vi "main.vi"() -> ()   [LabVIEW 2020]
doc: "Ce VI modèle est conçu pour le modèle de conception Gestionnaire de messages dans une file d'attente.\n\nLa boucle de gestion d'événements génère des messages en fonction des actions sur l'interface utilisateur.\n\nLa boucle de gestion de messages traite les messages générés par la boucle de gestion d'événements ou par d'autres messages. Les messages sont des valeurs chaîne ; il est donc facile d'ajouter de nouveaux messages à la structure condition Conditions de messages de la boucle de gestion de messages Chaque cluster Message peut en outre fournir une valeur optionnelle pour Données de message, un variant qui peut être converti aux données requises pour un message spécifique."
uses:
  controls/UI Data.ctl
  support/Message Queue/Enqueue Message (Single).vi
  <vilib>/Utility/error.llb/Error Cluster From Error Code.vi
  <vilib>/ErrorRing/Error Ring.xnode
  support/Message Queue/Message Queue.lvlib
  support/User Event - Stop/User Event - Stop.lvlib
  cDaqlib/cDaq.lvlib
panel:
  in  "Target position(°)":dbl
  in  "frequency (Hz)":i32 min=0 max=4000 step=1
  out "isHome?":bool
  in  "Tourner vers position":bool
  in  "Tourner en continue":bool
  out "ms for 1°":dbl
  out "passed ms":u32
  out "Position(°)":dbl
  out "AvgTimePerRev(s)":dbl
  out "temps(s)/tour (360°)":dbl[](array[numeric])
  in  "direction":bool
  out "enable = 0":i32
  out "tension compteur (V)":dbl
  out "DAQ HANDLE":u32
  out "Exit":bool
  out "compteur":i32
  out "Rotation status":bool
  in  "calibrer":bool
  in  "adresse":string
  out "Debug":string
  in  "deconnecter":bool
  in  "connecter":bool
  in  "Quitter":bool
  # "D'abord se connecter par USB à la carte DAQ. Si pas de nom préscisé le premier équipement disponible sera choisis."
  # "Passage devant\ndétecteur"
  # "Ferme proprement la connection avec la carte et libère les ressources."
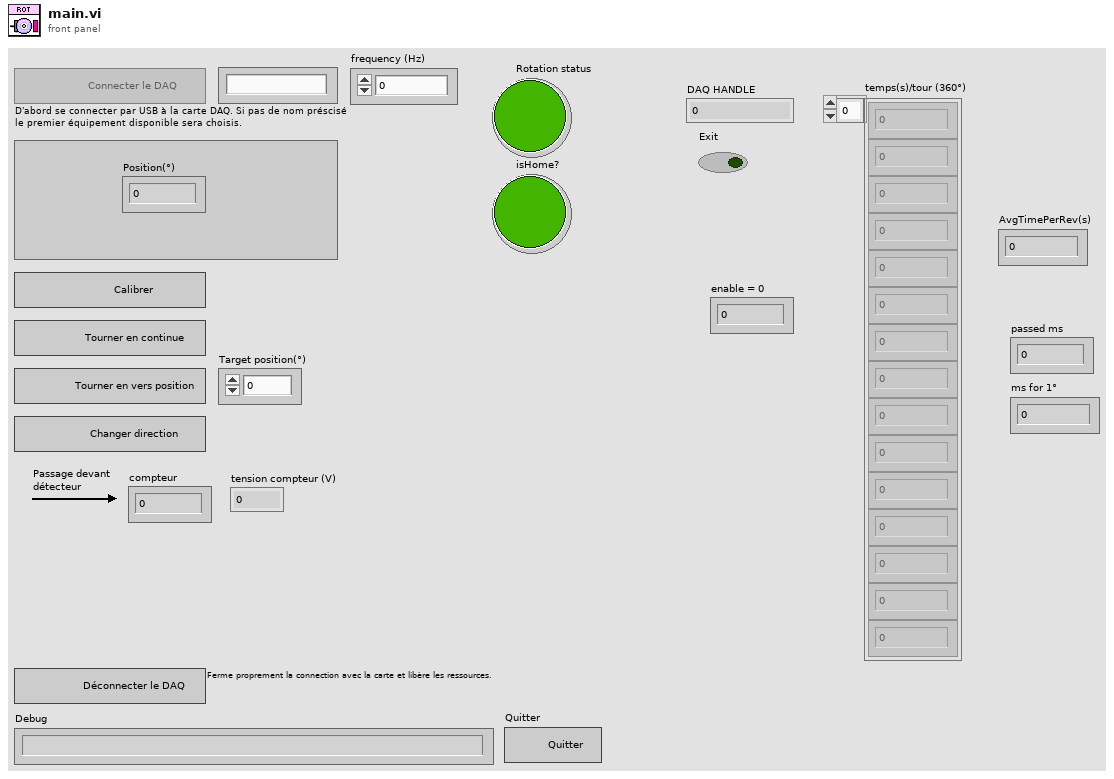
[diagram p1: front panel]
types:
  T1 = typedef "UI Data.ctl" = cluster{"Booléen <À remplacer>":bool, "Chaîne <À remplacer>":string, "Numérique <À remplacer>":dbl, "Réf. Action 1":refnum<vi>, "Réf. Action 2":refnum<vi>, "Réf. Affichage des données":refnum<vi>, "Réf du bouton Quitter":refnum<vi>, "DAQ handle":u32, "DAQ HANDLE ref":refnum<vi>, "frequency":refnum<vi>, "status":refnum<vi>, "Position(°)":refnum<vi>, "isHome?":refnum<vi>}
  T2 = cluster{"état":bool, "code":i32, "source":string}
  T3 = typedef "Message Queue.lvlib/All Message Queues.ctl" = cluster{"IU":refnum<queue>}
  T4 = enum8{"Enabled", "Disabled", "Disabled and Grayed Out"}
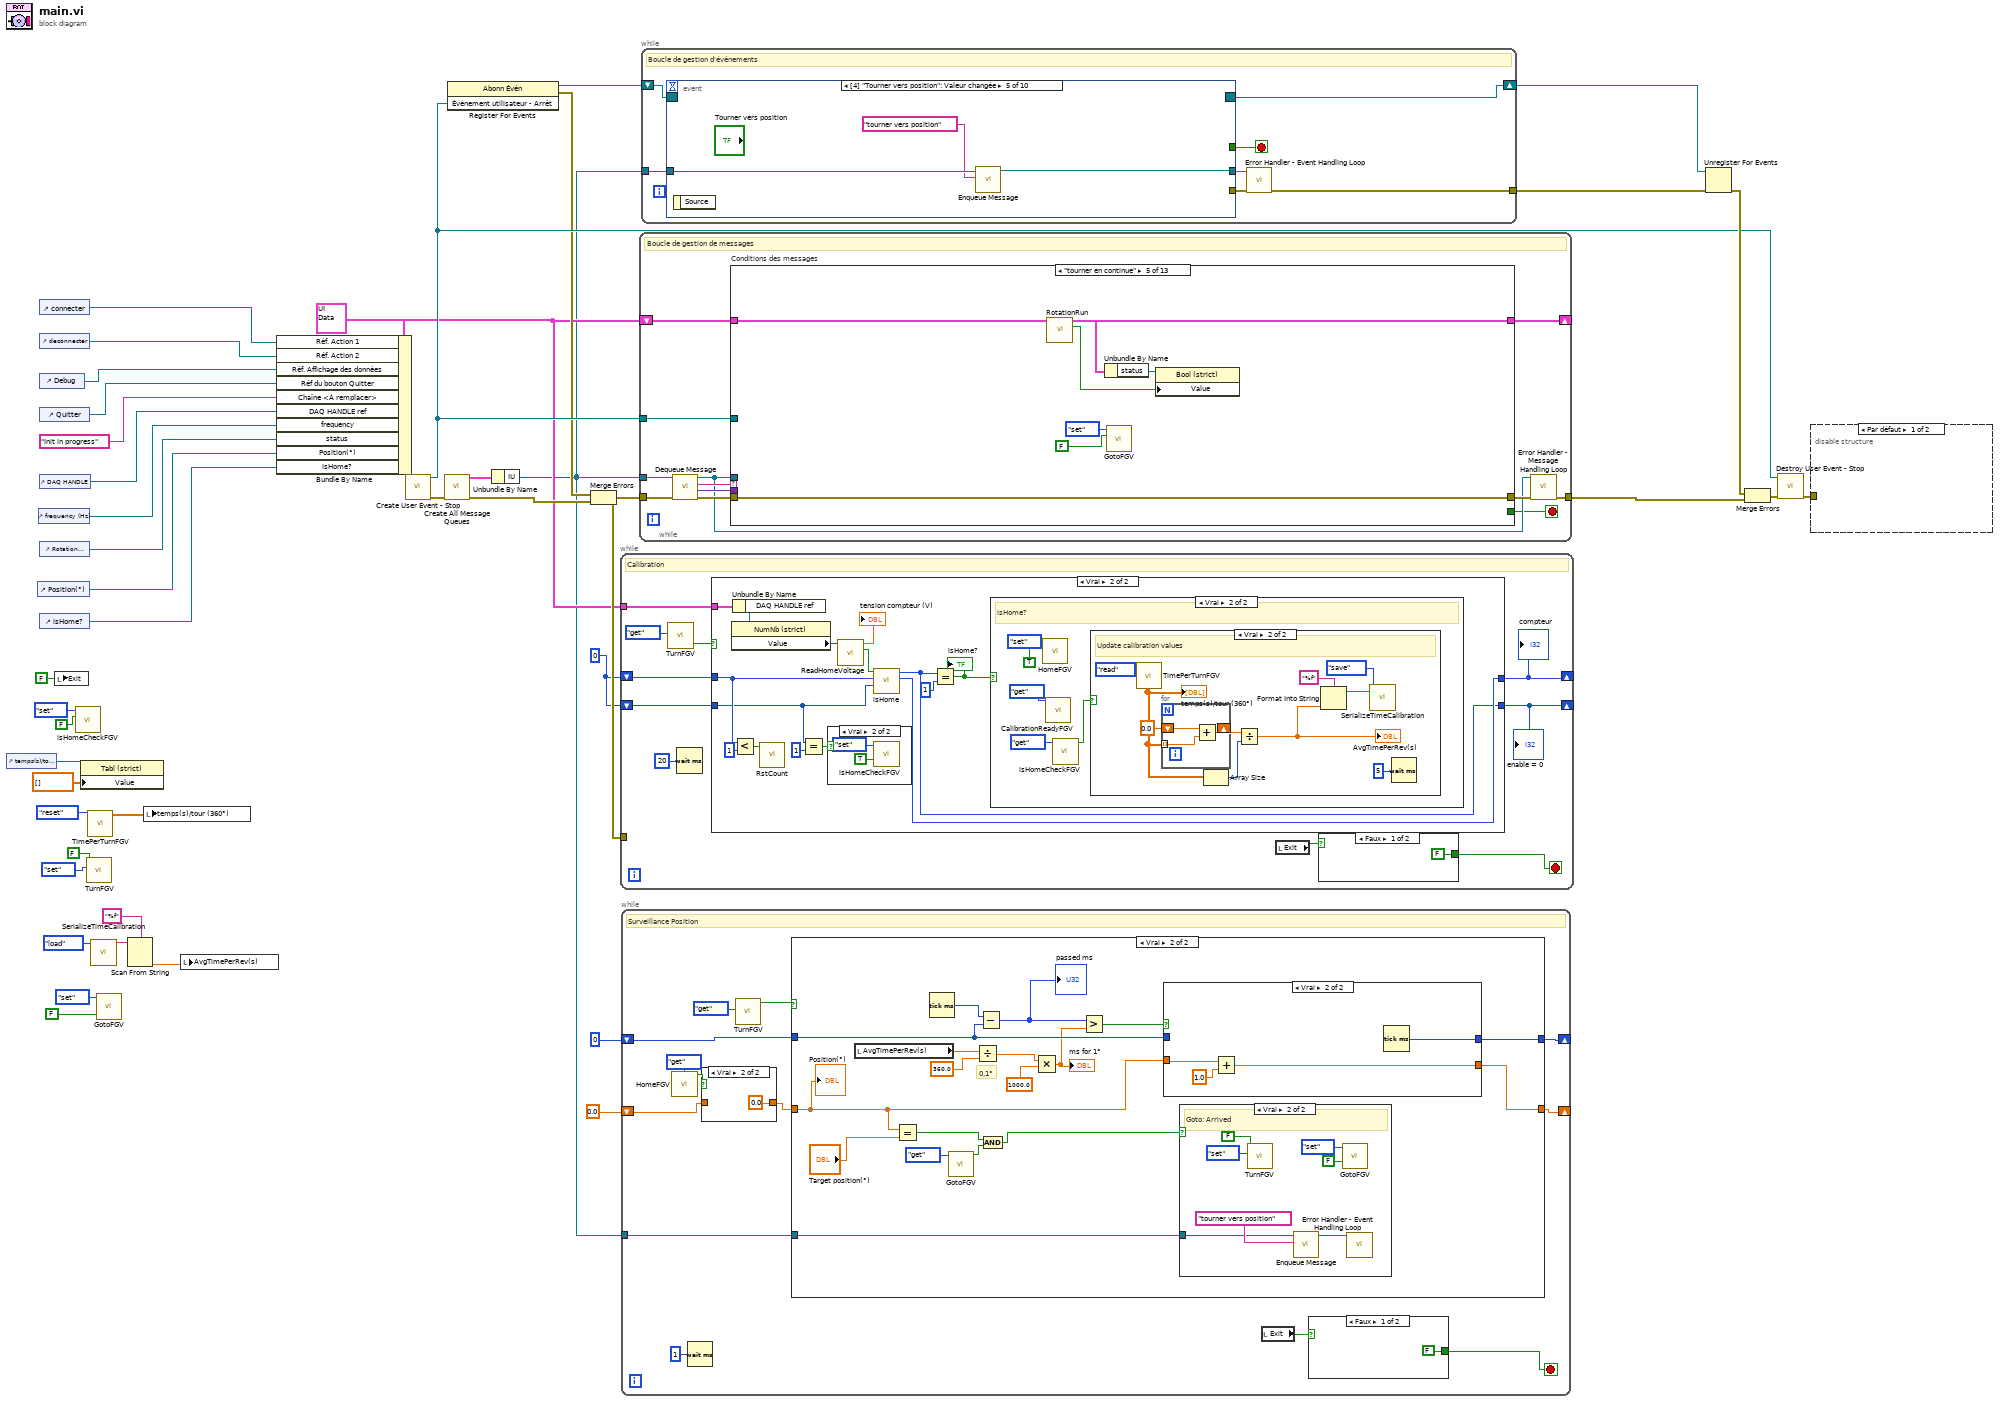
[diagram p0: block diagram]
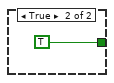
[diagram p3: hidden frame]
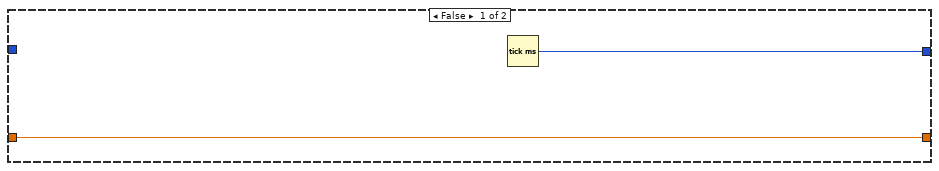
[diagram p4: hidden frame]
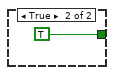
[diagram p7: hidden frame]
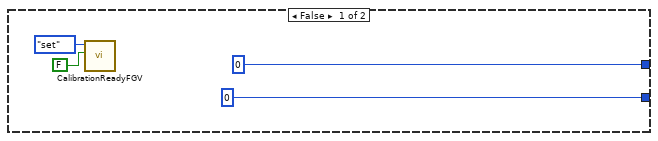
[diagram p8: hidden frame]
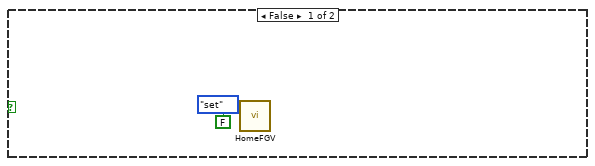
[diagram p10: hidden frame]
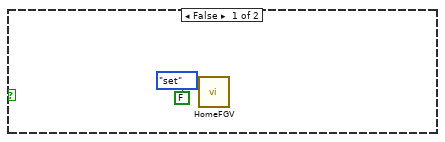
[diagram p11: hidden frame]
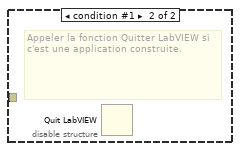
[diagram p12: hidden frame]
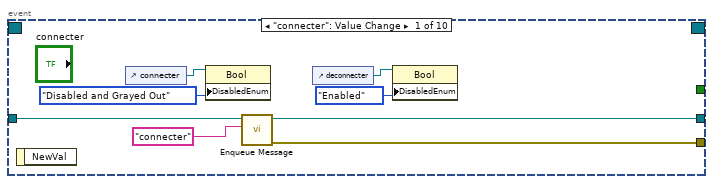
[diagram p13: hidden frame]
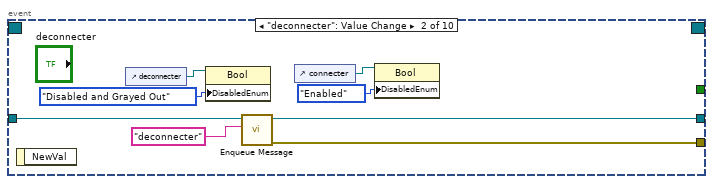
[diagram p14: hidden frame]
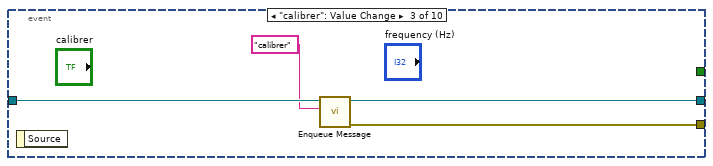
[diagram p15: hidden frame]
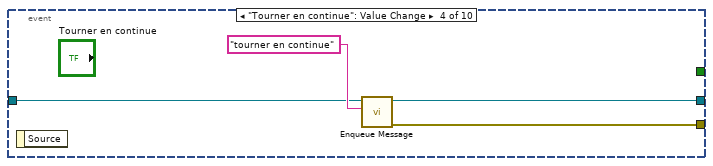
[diagram p16: hidden frame]
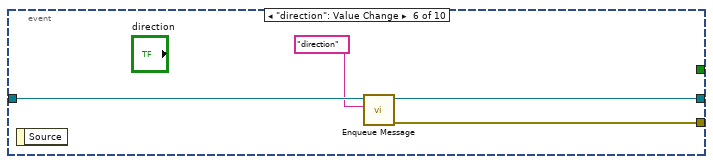
[diagram p17: hidden frame]
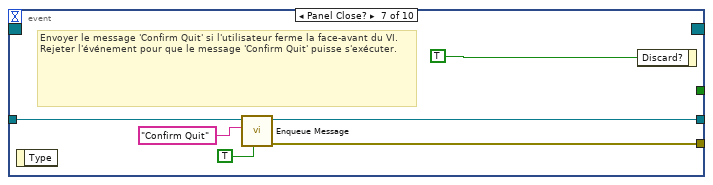
[diagram p18: hidden frame]
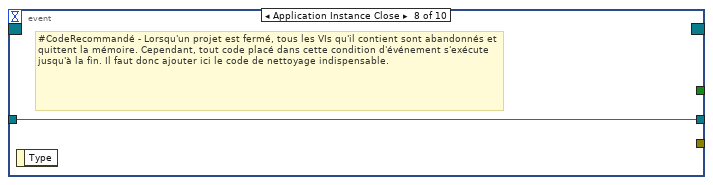
[diagram p19: hidden frame]
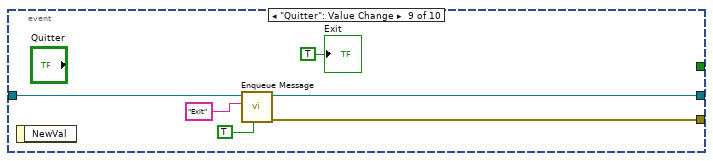
[diagram p20: hidden frame]
diagram:
  w22 = 0
  n1 = control-ref of="temps(s)/tour (360°)"() -> (w19:refnum<vi>)
  n2 = control-ref of="Position(°)"() -> (w9:refnum<vi>)
  n3 = control-ref of="frequency (Hz)"() -> (w4:refnum<vi>)
  n4 = control-ref of="connecter"() -> (w29:refnum<vi>)
  n5 = control-ref of="deconnecter"() -> (w30:refnum<vi>)
  n6 = control-ref of="Debug"() -> (w31:refnum<vi>)
  n7 = control-ref of="Quitter"() -> (w7:refnum<vi>)
  n8 = control-ref of="DAQ HANDLE"() -> (w10:refnum<vi>)
  n9 = control-ref of="Rotation status"() -> (w11:refnum<vi>)
  n10 = control-ref of="isHome?"() -> (w8:refnum<vi>)
  n11 = local write "Exit"(FALSE ("Exit")) -> ()
  n12 = call "isHomeCheckFGV.vi"("isHomeCheck?"=FALSE, "state"=enum16{"get", "set"}."set") -> ()  [unwired: 9 in, 1 out]
  n13 = property class="Tabl (strict)"(reference=w19, "Value"=dbl[] [] ("Valeur")) -> ()  [unwired: 1 in, 2 out]
  n14 = call "TurnFGV.vi"("Énum"=enum16{"set", "get"}."set", "set"=FALSE) -> ()  [unwired: 9 in, 1 out]
  n15 = call "TimePerTurnFGV.vi"("Énum"=enum16{"reset", "read", "home"}."reset") -> ("temps(s)/tour (360°)"=w16:dbl[])  [unwired: 9 in, 1 out]
  n16 = call "SerializeTimeCalibration.vi"("cmd"=enum16{"load", "save"}."load") -> ("TimeCalibration out"=w15:string)  [unwired: 10 in]
  n17 = call "GotoFGV.vi"("goto?"=FALSE, "goto pos"=enum16{"get", "set"}."set") -> ()  [unwired: 9 in, 1 out]
  n18 = Scan From String(format string="%f" ("chaîne de format"), input string=w15) -> (output 1=w12:dbl)  [unwired: 3 in, 3 out]
  n19 = local write "temps(s)/tour (360°)"(w16) -> ()
  n20 = local write "AvgTimePerRev(s)"(w12) -> ()
  n21 = Bundle By Name(cluster=T1 {"Booléen <À remplacer>"=FALSE, "Chaîne <À remplacer>"="", "Numérique <À remplacer>"=0.0, "Réf. Action 1"=refnum, "Réf. Action 2"=refnum, "Réf. Affichage des données"=refnum, "Réf du bouton Quitter"=refnum, "DAQ handle"=0, "DAQ HANDLE ref"=refnum, "frequency"=refnum, "status"=refnum, "Position(°)"=refnum, "isHome?"=refnum} ("Data Cluster"), "Réf. Action 1"=w29, "Réf. Action 2"=w30, "Réf. Affichage des données"=w31, "Réf du bouton Quitter"=w7, "Chaîne <À remplacer>"="Init in progress" ("Initial Message"), "DAQ HANDLE ref"=w10, "frequency"=w4, "status"=w11, "Position(°)"=w9, "isHome?"=w8) -> (w26:T1)
  n22 = call "Create User Event - Stop.vi"() -> ("error out"=w41:T2, "Événement utilisateur - Arrêt"=w34:refnum<user-event>)  [unwired: 10 in]
  n23 = call "Create All Message Queues.vi"("error in (no error)"=w41) -> ("error out"=w44:T2, "Files d'attente de messages en sortie"=w43:T3)  [unwired: 9 in]
  n24 = register-events(w34) -> (reference out=w35:refnum<event-registration>, error out=w33:errorcluster)  [unwired: 2 in]
  n25 = Unbundle By Name(w43) -> ("IU"=w1:refnum<queue>)
  n26 = Merge Errors(w33, w44) -> (w32:errorcluster)
  n27 = while {
    tunnel: w26 -> [w47]
    shift-right: [w50] -> _
    shift-left: w22 -> [w51]
    tunnel: w32 -> [_]
    shift-right: [w45] -> _
    shift-left: w22 -> [w46]
    stop <- w49 stop-if-true
    # "Calibration"
    n28 = call "TurnFGV.vi"("Énum"=enum16{"set", "get"}."get") -> ("get"=w53:bool)  [unwired: 10 in]
    n29 = Wait (ms)(milliseconds to wait=u32 20 ("attente (ms)")) -> ()  [unwired: 1 out]
    n30 = case shown="Vrai" w53 {
      tunnel: w47 -> [_ w75]
      tunnel: w51 -> [_ w62]
      tunnel: [0 w72] -> w50
      tunnel: w46 -> [_ w61]
      tunnel: [0 w65] -> w45
      frame False {
        n31 = call "CalibrationReadyFGV.vi"("Énum"=enum16{"get", "1stClk", "set"}."set", "set"=FALSE) -> ()  [unwired: 8 in, 1 out]
      }
      frame True {
        n32 = Unbundle By Name(w75) -> ("DAQ HANDLE ref"=w71:refnum<vi>)
        n33 = property class="NumNb (strict)"(reference=w71) -> ("Value"=w70:u32)  [unwired: 1 in, 2 out]
        n34 = Less?(x=w62, y=1) -> (x < y?=w67:bool)
        n35 = call "RstCount.vi"("Reset counter"=w67) -> ()  [unwired: 11 in]
        n36 = Equal?(x=w61, y=1) -> (x = y?=w63:bool)
        n37 = case shown="Vrai" w63 {
          frame False {
          }
          frame True {
            n38 = call "isHomeCheckFGV.vi"("isHomeCheck?"=TRUE, "state"=enum16{"get", "set"}."set") -> ()  [unwired: 9 in, 1 out]
          }
        }
        n39 = call "ReadHomeVoltage.vi"("Handle"=w70) -> ("At home"=w73:bool, "Voltage read 0V=in position"=→"tension compteur (V)":dbl)  [unwired: 9 in]
        n40 = call "isHome.vi"("HomeDetected last state"=w61, "Counter last state"=w62, "Home area detected"=w73) -> ("Counter"=w72:i32, "HomeDetected=1"=w65:i32)  [unwired: 7 in]
        n41 = Equal?(x=w65, y=1) -> (x = y?=w64:bool)
        "isHome?" <- w64
        n42 = case shown="Vrai" w64 {
          frame False {
            n43 = call "HomeFGV.vi"("Énum"=enum16{"set", "get"}."set", "Booléen"=FALSE) -> ()  [unwired: 8 in, 1 out]
          }
          frame True {
            # "isHome?"
            n44 = call "HomeFGV.vi"("Énum"=enum16{"set", "get"}."set", "Booléen"=TRUE) -> ()  [unwired: 8 in, 1 out]
            n45 = call "CalibrationReadyFGV.vi"("Énum"=enum16{"get", "1stClk", "set"}."get") -> ()  [unwired: 9 in, 1 out]
            n46 = call "isHomeCheckFGV.vi"("state"=enum16{"get", "set"}."get") -> ("HomeisCheck"=w81:bool)  [unwired: 10 in]
            n47 = case shown="Vrai" w81 {
              frame False {
                n48 = call "HomeFGV.vi"("Énum"=enum16{"set", "get"}."set", "Booléen"=FALSE) -> ()  [unwired: 8 in, 1 out]
              }
              frame True {
                # "Update calibration values"
                n49 = call "TimePerTurnFGV.vi"("Énum"=enum16{"reset", "read", "home"}."read") -> ("temps(s)/tour (360°)"=w95:dbl[])  [unwired: 9 in, 1 out]
                "temps(s)/tour (360°)" <- w95
                n50 = for {
                  tunnel: w95 -> [w98] mode=indexing
                  shift-right: [w97] -> w94
                  shift-left: 0.0 -> [w99]
                  n51 = Add(x=w99, y=w98) -> (x+y=w97:dbl)
                }
                n52 = Array Size(array=w95) -> (size(s)=w93:i32)
                n53 = Divide(x=w94, y=w93) -> (x/y=w88:dbl)
                "AvgTimePerRev(s)" <- w88
                n54 = Format Into String(format string="%f" ("chaîne de format"), w88) -> (resulting string=w89:string)  [unwired: 2 in, 1 out]
                n55 = call "SerializeTimeCalibration.vi"("TimeCalibration in"=w89, "cmd"=enum16{"load", "save"}."save") -> ()  [unwired: 9 in, 1 out]
                n56 = Wait (ms)(milliseconds to wait=u32 5 ("attente (ms)")) -> ()  [unwired: 1 out]
              }
            }
          }
        }
      }
    }
    "compteur" <- w50
    "enable = 0" <- w45
    n57 = local read "Exit"() -> (w48:bool)
    n58 = case shown="Faux" w48 {
      tunnel: [FALSE TRUE] -> w49
      frame False {
      }
      frame True {
      }
    }
  }
  n59 = while {
    shift-right: [w109] -> _
    shift-left: u32 0 ("millisecond timer value") -> [w112]
    shift-right: [w108] -> _
    shift-left: 0.0 -> [w104]
    tunnel: w1 -> [w100]
    stop <- w111 stop-if-true
    # "Surveillance Position"
    n60 = call "HomeFGV.vi"("Énum"=enum16{"set", "get"}."get") -> ("home ?"=w106:bool)  [unwired: 9 in]
    n61 = Wait (ms)(milliseconds to wait=u32 1 ("attente (ms)")) -> ()  [unwired: 1 out]
    n62 = case shown="Vrai" w106 {
      tunnel: w104 -> [w113 _]
      tunnel: [w113 0.0] -> w103
      frame False {
      }
      frame True {
      }
    }
    n63 = call "TurnFGV.vi"("Énum"=enum16{"set", "get"}."get") -> ("get"=w101:bool)  [unwired: 10 in]
    n64 = case shown="Vrai" w101 {
      tunnel: w112 -> [_ w131]
      tunnel: [w118 w130] -> w109
      tunnel: w103 -> [w117 w125]
      tunnel: [w117 w132] -> w108
      tunnel: w100 -> [_ w119]
      frame False {
        n65 = Tick Count (ms)() -> (millisecond timer value=w118:u32)
      }
      frame True {
        # "0,1°"
        n66 = local read "AvgTimePerRev(s)"() -> (w135:dbl)
        n67 = Equal?(x=w125, y="Target position(°)") -> (x = y?=w123:bool)
        n68 = Tick Count (ms)() -> (millisecond timer value=w136:u32)
        n69 = call "GotoFGV.vi"("goto pos"=enum16{"get", "set"}."get") -> ("moving to position"=w121:bool)  [unwired: 10 in]
        n70 = Divide(x=w135, y=360.0) -> (x/y=w129:dbl)
        n71 = Subtract(x=w136, y=w131) -> (x-y=w126:u32)
        "passed ms" <- w126
        n72 = And(x=w123, y=w121) -> (x .and. y?=w120:bool)
        n73 = Multiply(x=w129, y=1000.0) -> (x*y=w127:dbl)
        "ms for 1°" <- w127
        n74 = Greater?(x=w126, y=w127) -> (0:w133:bool)
        n75 = case shown="Vrai" w133 {
          tunnel: w125 -> [w145 w149]
          tunnel: [w145 w146] -> w132
          tunnel: w131 -> [w144 _]
          tunnel: [w144 w147] -> w130
          frame False {
          }
          frame True {
            n76 = Add(x=w149, y=1.0) -> (x+y=w146:dbl)
            n77 = Tick Count (ms)() -> (millisecond timer value=w147:u32)
          }
        }
        n78 = case shown="Vrai" w120 {
          tunnel: w119 -> [_ w137]
          frame False {
          }
          frame True {
            # "Goto: Arrived"
            n79 = call "TurnFGV.vi"("Énum"=enum16{"set", "get"}."set", "set"=FALSE) -> ()  [unwired: 9 in, 1 out]
            n80 = call-poly "Enqueue Message.vi"("Message"="tourner vers position", "File d'attente de messages"=w137) -> ("File d'attente de message dup."=w139:refnum<queue>)  [unwired: 8 in, 1 out]
            n81 = call "GotoFGV.vi"("goto?"=FALSE, "goto pos"=enum16{"get", "set"}."set") -> ()  [unwired: 9 in, 1 out]
            n82 = call "Error Handler - Event Handling Loop.vi"("File d'attente de messages"=w139) -> ()  [unwired: 9 in, 2 out]
          }
        }
        "Position(°)" <- w125
      }
    }
    n83 = local read "Exit"() -> (w110:bool)
    n84 = case shown="Faux" w110 {
      tunnel: [FALSE TRUE] -> w111
      frame False {
      }
      frame True {
      }
    }
  }
  n85 = while {
    tunnel: w1 -> [w154]
    shift-right: [w160] -> _
    shift-left: w26 -> [w161]
    tunnel: w34 -> [w159]
    tunnel: w32 -> [w158]
    tunnel: [w153] -> w42
    stop <- w150 stop-if-true
    # "Boucle de gestion de messages"
    n86 = call "Dequeue Message.vi"("error in (no error)"=w158, "File d'attente de messages"=w154) -> ("error out"=w157:T2, "Données de message"=w155:variant, "Message"=w156:string, "File d'attente de message dup."=w151:refnum<queue>)  [unwired: 6 in]
    n87 = case "Conditions des messages" shown="\"tourner en continue\"" w156 {
      selector: w156 -> [_ _ _ _ _ _ _ _ _ _ _ _ w289]
      tunnel: w151 -> [w176 w191 w212 _ _ _ _ _ _ w263 _ w287 _]
      tunnel: w157 -> [w178 w192 w214 w224 w231 w238 w246 w251 w260 w267 w270 w281 _]
      tunnel: [w179 w193 w215 w224 w231 w238 w246 w252 w254 w265 w268 w284 w290] -> w152
      tunnel: w161 -> [w168 w180 w207 w220 w230 w236 w245 w253 w259 w266 w269 w274 w291]
      tunnel: [w168 w181 w207 w222 w227 w234 w245 w253 w259 w266 w269 w274 w291] -> w160
      tunnel: [_ _ _ _ _ _ _ _ _ _ _ TRUE _] -> w150
      tunnel: w155 -> [_ _ _ _ _ _ _ w250 w258 _ _ w278 _]
      tunnel: w159 -> [_ _ _ _ _ _ _ _ _ _ _ w283 _]
      frame "Initialize" {
        # "Initialize - Toute la tâche d'initialisation doit se faire dans ce message puisque les autres boucles risquent d'ajouter des messages qui s'exécutent juste après celui-ci à la file."
        n88 = control-ref of="Rotation status"() -> (w175:refnum<vi>)
        n89 = control-ref of="connecter"() -> (w173:refnum<vi>)
        n90 = control-ref of="deconnecter"() -> (w174:refnum<vi>)
        n91 = property class="Bool (strict)"(reference=w175, "DisabledEnum"=T4."Disabled" ("Désactivé")) -> ()  [unwired: 1 in, 2 out]
        n92 = property class="Bool"(reference=w173, "DisabledEnum"=T4."Enabled" ("Désactivé")) -> ()  [unwired: 1 in, 2 out]
        n93 = property class="Bool"(reference=w174, "DisabledEnum"=T4."Disabled and Grayed Out" ("Désactivé")) -> ()  [unwired: 1 in, 2 out]
        n94 = Unbundle By Name(w168) -> ("status"=w167:refnum<vi>, "isHome?"=w164:refnum<vi>, "DAQ HANDLE ref"=w163:refnum<vi>)
        n95 = call-poly "Enqueue Message.vi"("error in (no error)"=w178, "Données de message"="initialize" ("Message"), "Message"="Update Display", "File d'attente de messages"=w176) -> ("error out"=w179:T2)  [unwired: 6 in, 1 out]
        n96 = property class="NumNb (strict)"(reference=w163, "Value"=u32 0 ("Valeur")) -> ()  [unwired: 1 in, 2 out]
        n97 = property class="Bool (strict)"(reference=w167, "Value"=FALSE ("Valeur")) -> ()  [unwired: 1 in, 2 out]
        n98 = property class="Bool (strict)"(reference=w164, "Value"=FALSE ("Valeur")) -> ()  [unwired: 1 in, 2 out]
      }
      frame "connecter" {
        w186 = "Update Display" ("Message")
        # "Appel la DLL pour se connecter au DAQ"
        n99 = call "createDAQ.vi"("device"="adresse") -> ("function return"=w184:u32)  [unwired: 9 in]
        "DAQ HANDLE" <- w184
        n100 = call-poly "Enqueue Message.vi"("error in (no error)"=w192, "Données de message"="Demande de connection" ("\"Do Something\" button pressed"), "Message"=w186, "File d'attente de messages"=w191) -> ("error out"=w188:T2, "File d'attente de message dup."=w189:refnum<queue>)  [unwired: 6 in]
        n101 = Not Equal?(x=w184, y=u32 0) -> (x != y?=w182:bool)
        n102 = case shown="Vrai" w182 {
          tunnel: w189 -> [_ w203]
          tunnel: w188 -> [_ w202]
          tunnel: [T2 {"état"=TRUE, "code"=0, "source"="Erreur de connection"} ("error out") w201] -> w187
          tunnel: w186 -> [_ w200]
          tunnel: w180 -> [w195 w198]
          tunnel: w184 -> [_ w197]
          tunnel: [w195 w196] -> w181
          frame False {
          }
          frame True {
            n103 = Bundle By Name(cluster=w198, "DAQ handle"=w197) -> (w196:T1)
            n104 = call-poly "Enqueue Message.vi"("error in (no error)"=w202, "Données de message"="Connecté" ("\"Do Something\" button pressed"), "Message"=w200, "File d'attente de messages"=w203) -> ("error out"=w201:T2)  [unwired: 6 in, 1 out]
          }
        }
        n105 = Merge Errors(w187) -> (w193:errorcluster)
      }
      frame "deconnecter" {
        # "Libère les ressources"
        n106 = Unbundle By Name(w207) -> ("DAQ HANDLE ref"=w206:refnum<vi>)
        n107 = property class="NumNb (strict)"(reference=w206) -> ("Value"=w208:u32)  [unwired: 1 in, 2 out]
        n108 = call "destroyDAQ.vi"("handle"=w208) -> ("Succés?"=w209:bool)  [unwired: 10 in]
        n109 = case shown="Vrai" w209 {
          tunnel: w206 -> [_ w217]
          frame False {
          }
          frame True {
            n110 = property class="NumNb (strict)"(reference=w217, "Value"=u32 0 ("DAQ handle")) -> ()  [unwired: 1 in, 2 out]
          }
        }
        n111 = call-poly "Enqueue Message.vi"("error in (no error)"=w214, "Données de message"="DAQ déconnecté" ("\"Do Something Else\" button pressed"), "Message"="Update Display", "File d'attente de messages"=w212) -> ("error out"=w213:T2)  [unwired: 6 in, 1 out]
        n112 = Merge Errors(w213) -> (w215:errorcluster)
        n113 = call "TurnFGV.vi"("Énum"=enum16{"set", "get"}."set", "set"=FALSE) -> ()  [unwired: 9 in, 1 out]
      }
      frame "calibrer" {
        n114 = call "GotoFGV.vi"("goto?"=FALSE, "goto pos"=enum16{"get", "set"}."set") -> ()  [unwired: 9 in, 1 out]
        n115 = call "RotationRun.vi"("Data Cluster en entrée"=w220) -> ("Booléen"=→"Rotation status":bool, "Data Cluster en sortie"=w222:T1)  [unwired: 9 in]
        n116 = call "CalibrationStart.vi"("Booléen"=TRUE) -> ()  [unwired: 11 in]
      }
      frame "tourner en continue" {
        n117 = call "RotationRun.vi"("Data Cluster en entrée"=w230) -> ("Booléen"=w228:bool, "Data Cluster en sortie"=w227:T1)  [unwired: 9 in]
        n118 = Unbundle By Name(w230) -> ("status"=w229:refnum<vi>)
        n119 = call "GotoFGV.vi"("goto?"=FALSE, "goto pos"=enum16{"get", "set"}."set") -> ()  [unwired: 9 in, 1 out]
        n120 = property class="Bool (strict)"(reference=w229, "Value"=w228) -> ()  [unwired: 1 in, 2 out]
      }
      frame "tourner vers position" {
        n121 = call "GotoFGV.vi"("goto?"=TRUE, "goto pos"=enum16{"get", "set"}."set") -> ()  [unwired: 9 in, 1 out]
        n122 = call "RotationRun.vi"("Data Cluster en entrée"=w236) -> ("Booléen"=w235:bool, "Data Cluster en sortie"=w234:T1)  [unwired: 9 in]
        n123 = Unbundle By Name(w236) -> ("status"=w237:refnum<vi>)
        n124 = property class="Bool (strict)"(reference=w237, "Value"=w235) -> ()  [unwired: 1 in, 2 out]
      }
      frame "direction" {
        # "Inverser à chaque clic"
        n125 = Unbundle By Name(w245) -> ("DAQ HANDLE ref"=w244:refnum<vi>)
        n126 = property class="NumNb (strict)"(reference=w244) -> ("Value"=w240:u32)  [unwired: 1 in, 2 out]
        n127 = feedback #1(TRUE) -> (w241:bool)
        n128 = call "Direction.vi"("pin"=1, "handle"=w240, "Direction?"=w241) -> ()  [unwired: 8 in, 1 out]
        n129 = Not(x=w241) -> (.not. x?=w242:bool)
        n130 = feedback-in #1(w242) -> ()
      }
      frame "Update Display" {
        # "#CodeRecommandé - Pour séparer la boucle de gestion de messages de l'interface utilisateur, envisagez de créer des événements utilisateur (comme l'événement \"Arrêt\" de ce VI) pour envoyer des messages à la boucle de gestion d'événements quand l'interface utilisateur doit être mise à jour."
        # "Update Display - Convertir les données du message en chaîne pour l'afficher dans l'indicateur Affichage des données."
        n131 = Variant To Data(error in=w251, type="", Variant=w250) -> (data=→"Debug":string, error out=w248:errorcluster)
        n132 = Merge Errors(w248) -> (w252:errorcluster)
      }
      frame "Error" {
        # "#CodeRecommandé - Si vous changez le nom de ce message \"Error\" ici, vous devrez aussi le changer dans le VI Check Loop Error.vi."
        # "#CodeRecommandé - Envisagez de créer un système pour enregistrer les erreurs d'une façon ou d'une autre. Ces erreurs sont uniquement destinées aux notifications. La gestion d'erreurs spécifiques devrait se faire dans les conditons de messages qui ont générées l'erreur."
        # "Error - Afficher une boîte de dialogue d'erreur. Ce message est envoyé par les VIs \"Error Handler\" à la fin de l'exécution de chaque boucle de cette application."
        n133 = Variant To Data(error in=w260, type=errorcluster {"status"=FALSE, "code"=0, "source"=""} ("error constant"), Variant=w258) -> (data=w256:errorcluster, error out=w255:errorcluster)
        n134 = call <vilib>:"Simple Error Handler.vi"("error in (no error)"=w256) -> ()  [unwired: 4 in, 5 out]
        n135 = Merge Errors(w255) -> (w254:errorcluster)
      }
      frame "Confirm Quit" {
        # "#CodeNécessaire - Si vous voulez afficher une boîte de dialogue de confirmation (ou un autre message) avant de quitter l'application, placez le code ici. En général, ce message est envoyé à partir d'un événement Fermeture de face-avant ?"
        # "Confirm Quit - Message qui confirme si l'utilisateur voulait vraiment quitter l'application."
        n136 = call-poly "Enqueue Message.vi"("Message prioritaire ? (F)"=TRUE ("Priority Message? (F)"), "error in (no error)"=w267, "Message"="Exit", "File d'attente de messages"=w263) -> ("error out"=w264:T2)  [unwired: 6 in, 1 out]
        n137 = Merge Errors(w264) -> (w265:errorcluster)
      }
      frame "---Copy This Frame---" {
        # "Dupliquez cette étape pour créer de nouveaux messages.  Changez ce commentaire dans l'étape dupliquée pour décrire ce message."
        n138 = Merge Errors(w270) -> (w268:errorcluster)
      }
      frame "Exit" {
        # "Arrêter le VI"
        # "Libérer la référence à la file d'attente de messages"
        # "Exit - Quitter l'application."
        n139 = Unbundle By Name(w274) -> ("DAQ HANDLE ref"=w277:refnum<vi>)
        n140 = Variant To Data(type=errorcluster {"status"=FALSE, "code"=0, "source"=""} ("error constant"), Variant=w278) -> (data=w279:errorcluster)  [unwired: 1 in, 1 out]
        n141 = call <vilib>:"Simple Error Handler.vi"("error in (no error)"=w279) -> ()  [unwired: 4 in, 5 out]
        n142 = call "TurnFGV.vi"("Énum"=enum16{"set", "get"}."set", "set"=FALSE) -> ()  [unwired: 9 in, 1 out]
        n143 = property class="NumNb (strict)"(reference=w277) -> ("Value"=w273:u32)  [unwired: 1 in, 2 out]
        n144 = call "Fire User Event - Stop.vi"("Événement utilisateur - Arrêt"=w283) -> ("error out"=w282:T2)  [unwired: 10 in]
        n145 = Release Queue(queue=w287, error in (no error)=w281) -> (error out=w285:errorcluster)  [unwired: 1 in, 2 out]
        n146 = Not Equal?(x=w273, y=u32 0) -> (x != y?=w275:bool)
        n147 = case shown="Vrai" w275 {
          tunnel: w273 -> [_ w288]
          frame False {
          }
          frame True {
            # "#Clean Daq if not done before"
            n148 = call "destroy c Daq .vi"("handle"=w288) -> ()  [unwired: 9 in, 2 out]
          }
        }
        n149 = Merge Errors(w282, w285) -> (w284:errorcluster)
      }
      frame Default {
        # "La condition 'Par défaut' ne s'exécute que s'il y a un message qui n'est défini dans aucune des autres conditions.  Renvoyer une erreur de programmation."
        n150 = xnode ("Error Ring")("paramètre 0"=w289) -> ("sortie d'erreur"=w290:errorcluster)
      }
    }
    n151 = call "Error Handler - Message Handling Loop.vi"("error in (no error)"=w152, "File d'attente de messages"=w151) -> ("erreur en entrée dup."=w153:T2)  [unwired: 8 in, 1 out]
  }
  n152 = while {
    tunnel: w1 -> [w305]
    shift-right: [w303] -> w38
    shift-left: w35 -> [w304]
    tunnel: [w299] -> w36
    stop <- w301 stop-if-true
    # "Boucle de gestion d'événements"
    n153 = event shown="[4] \"Tourner vers position\": Valeur changée" {
      selector: w304 -> [_ _ _ _ _ _ _ _ _ _]
      dyn-events: [_ _ _ _ _ _ _ _ _ _] -> w303
      timeout: _ -> [_ _ _ _ _ _ _ _ _ _]
      tunnel: [_ _ _ _ _ _ _ _ _ TRUE ("Discard?")] -> w301
      tunnel: w305 -> [w313 w321 w324 w328 w332 w336 w341 w343 w349 w352]
      tunnel: [w310 w318 w325 w326 _ w334 w340 _ w348 _] -> w302
      tunnel: [w312 w320 w323 w327 w331 w335 w339 w343 w347 w352] -> w300
      event "connecter": Value Change {
        n154 = event-data() -> ()  [unwired: 1 in, 1 out]
        n155 = control-ref of="connecter"() -> (w306:refnum<vi>)
        n156 = property class="Bool"(reference=w306, "DisabledEnum"=T4."Disabled and Grayed Out" ("Désactivé")) -> ()  [unwired: 1 in, 2 out]
        n157 = call-poly "Enqueue Message.vi"("Message"="connecter", "File d'attente de messages"=w313) -> ("error out"=w310:T2, "File d'attente de message dup."=w312:refnum<queue>)  [unwired: 8 in]
        n158 = control-ref of="deconnecter"() -> (w309:refnum<vi>)
        n159 = property class="Bool"(reference=w309, "DisabledEnum"=T4."Enabled" ("Désactivé")) -> ()  [unwired: 1 in, 2 out]
      }
      event "deconnecter": Value Change {
        n160 = event-data() -> ()  [unwired: 1 in, 1 out]
        n161 = control-ref of="deconnecter"() -> (w317:refnum<vi>)
        n162 = property class="Bool"(reference=w317, "DisabledEnum"=T4."Disabled and Grayed Out" ("Désactivé")) -> ()  [unwired: 1 in, 2 out]
        n163 = call-poly "Enqueue Message.vi"("Message"="deconnecter", "File d'attente de messages"=w321) -> ("error out"=w318:T2, "File d'attente de message dup."=w320:refnum<queue>)  [unwired: 8 in]
        n164 = control-ref of="connecter"() -> (w314:refnum<vi>)
        n165 = property class="Bool"(reference=w314, "DisabledEnum"=T4."Enabled" ("Désactivé")) -> ()  [unwired: 1 in, 2 out]
      }
      event "calibrer": Value Change {
        n166 = event-data() -> ()  [unwired: 1 in, 1 out]
        n167 = call-poly "Enqueue Message.vi"("Message"="calibrer", "File d'attente de messages"=w324) -> ("error out"=w325:T2, "File d'attente de message dup."=w323:refnum<queue>)  [unwired: 8 in]
      }
      event "Tourner en continue": Value Change {
        n168 = event-data() -> ()  [unwired: 1 in, 1 out]
        n169 = call-poly "Enqueue Message.vi"("Message"="tourner en continue", "File d'attente de messages"=w328) -> ("error out"=w326:T2, "File d'attente de message dup."=w327:refnum<queue>)  [unwired: 8 in]
      }
      event "Tourner vers position": Value Change {
        n170 = event-data() -> ()  [unwired: 1 in, 1 out]
        n171 = call-poly "Enqueue Message.vi"("Message"="tourner vers position", "File d'attente de messages"=w332) -> ("File d'attente de message dup."=w331:refnum<queue>)  [unwired: 8 in, 1 out]
      }
      event "direction": Value Change {
        n172 = event-data() -> ()  [unwired: 1 in, 1 out]
        n173 = call-poly "Enqueue Message.vi"("Message"="direction", "File d'attente de messages"=w336) -> ("error out"=w334:T2, "File d'attente de message dup."=w335:refnum<queue>)  [unwired: 8 in]
      }
      event Panel Close? {
        # "Envoyer le message 'Confirm Quit' si l'utilisateur ferme la face-avant du VI. Rejeter l'événement pour que le message 'Confirm Quit' puisse s'exécuter."
        n174 = event-data() -> ()  [unwired: 1 in, 1 out]
        n175 = call-poly "Enqueue Message.vi"("Message prioritaire ? (F)"=TRUE ("Priority Message? (F)"), "Message"="Confirm Quit", "File d'attente de messages"=w341) -> ("error out"=w340:T2, "File d'attente de message dup."=w339:refnum<queue>)  [unwired: 7 in]
        n176 = event-data ("Event Filter Node")("Discard?"=TRUE) -> ()  [unwired: 1 in, 1 out]
      }
      event Application Instance Close {
        # "#CodeRecommandé - Lorsqu'un projet est fermé, tous les VIs qu'il contient sont abandonnés et quittent la mémoire. Cependant, tout code placé dans cette condition d'événement s'exécute jusqu'à la fin. Il faut donc ajouter ici le code de nettoyage indispensable."
        n177 = event-data() -> ()  [unwired: 1 in, 1 out]
      }
      event "Quitter": Value Change {
        n178 = event-data() -> ()  [unwired: 1 in, 1 out]
        n179 = call-poly "Enqueue Message.vi"("Message prioritaire ? (F)"=TRUE ("Priority Message? (F)"), "Message"="Exit", "File d'attente de messages"=w349) -> ("error out"=w348:T2, "File d'attente de message dup."=w347:refnum<queue>)  [unwired: 7 in]
        "Exit" <- TRUE ("Exit")
      }
      event User Event {
        # "La boucle de gestion de messages a traité un message \"Exit\", ce qui a déclenché cet événement pour arrêter la boucle de gestion d'événements."
        n180 = event-data() -> ()  [unwired: 1 in, 1 out]
        n181 = local write "Debug"("Quit called" ("Debug")) -> ()
      }
    }
    n182 = call "Error Handler - Event Handling Loop.vi"("error in (no error)"=w302, "File d'attente de messages"=w300) -> ("erreur en entrée dup."=w299:T2)  [unwired: 8 in, 1 out]
  }
  n183 = Unregister For Events(event registration refnum=w38, error in=w36) -> (error out=w39:errorcluster)
  n184 = Merge Errors(w39, w42) -> (w40:errorcluster)
  n185 = call "Destroy User Event - Stop.vi"("error in (no error)"=w40, "Événement utilisateur - Arrêt"=w34) -> ("error out"=w37:T2)  [unwired: 9 in]
  n186 = disable-structure "Conditional Disable Structure" shown="Par défaut" {
    disable-tunnel: w37 -> [_ _]
    frame condition #0 (active) {
    }
    frame condition #1 {
      # "Appeler la fonction Quitter LabVIEW si c'est une application construite."
      n187 = Quit LabVIEW() -> ()  [unwired: 1 in]
    }
  }
